vi "prova.vi"() -> ()   [LabVIEW 2021]
uses:
  <vilib>/MakerHub/LINX/Public/Peripherals/Analog/Analog Read 1 Chan.vi
  <vilib>/MakerHub/LINX/Public/Peripherals/Analog/Analog Read N Chans.vi
  <vilib>/MakerHub/LINX/Private/Local IO/LinxAnalogRead.vi
  <vilib>/MakerHub/LINX/Public/Utilities/Check Channel.vi
  <vilib>/Utility/file.llb/Write Delimited Spreadsheet (DBL).vi
  <vilib>/MakerHub/LINX/Public/Utilities/Open Serial.vi
  <vilib>/MakerHub/LINX/Public/Sensors/Motion/Servo/Servo Open One Channel.vi
  <vilib>/MakerHub/LINX/Public/Sensors/Motion/Servo/Servo Set Pulse Width One Channel.vi
  <vilib>/MakerHub/LINX/Private/Utilties/Generate Error.vi
  <vilib>/MakerHub/LINX/Public/Sensors/Motion/Servo/Servo Close One Channel.vi
  <vilib>/Utility/file.llb/Read Delimited Spreadsheet (DBL).vi
  <vilib>/MakerHub/LINX/LMH-LINX.lvlib
  <vilib>/MakerHub/LINX/Public/Sensors/Motion/Servo/Servo.lvlib
panel:
  out "Average":dbl[](array[numeric])
  out "Min. Wert":dbl
  out "Max. Wert":dbl
  out "all rows":dbl[][](array[numeric]) caption="Alle Zeilen"
  in  "Retrieve":bool
  in  "Dateipfad (Dialog verwenden)":path=path "C:/Users/Lucas Gomes/Documents/teste"
  in  "Button Channel":u8=2
  in  "Temp Channel":u8
  in  "Servo Channel":u8=3
  in  "VISA-Referenz (Eingang)":refnum<visa-resource-name>="COM3"
  in  "Stopp-Schaltfläche":bool
  out "Thermometer":dbl(slide) scale=0.0..100.0
  out "Signalverlaufsdiagramm 2":dbl(graph)
  # "5"
  # "Past data"
  # "Configurations"
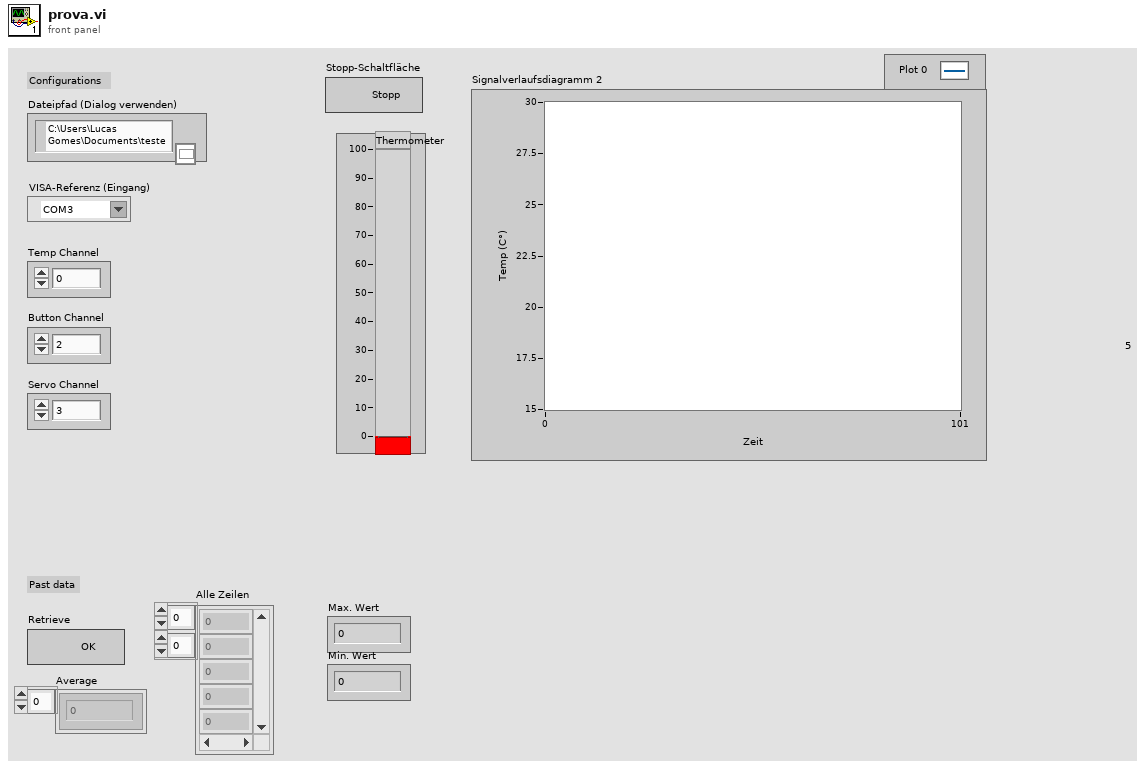
[diagram p1: front panel]
types:
  T1 = typedef "LMH-LINX.lvlib/LINX Ref.ctl" = cluster{"IO":T2, "Interface":T3, "LINX Device Config":T4}
  T2 = typedef "LMH-LINX.lvlib/Platform.ctl" = enum16{"Remote", "Local"}
  T3 = typedef "LMH-LINX.lvlib/Interface.ctl" = enum16{"Serial", "TCP"}
  T4 = typedef "LMH-LINX.lvlib/Device.lvlib/LINX Device Config.ctl" = cluster{"Interface":T3, "COM Port":refnum<visa-resource-name>, "TCP Configuration":T5, "Device Family":u8, "Device ID":u8, "Device Name":string, "TCP Ref":refnum<k5>, "Channels":T6}
  T5 = typedef "LMH-LINX.lvlib/Device.lvlib/TCP Config.ctl" = cluster{"IP Address":string, "Port":u16}
  T6 = typedef "LMH-LINX.lvlib/Channels.ctl" = cluster{"DI":u8[], "DO":u8[], "AI":u8[], "AO":u8[], "PWM":u8[], "QE":u8[], "UART":u8[], "I2C 2":u8[], "SPI":u8[], "CAN":u8[], "Servo":u8[], "AI Ref (V)":dbl, "AI Resolution (Bits)":u8, "AO Ref (V)":dbl, "AO Resolution (Bits)":u8}
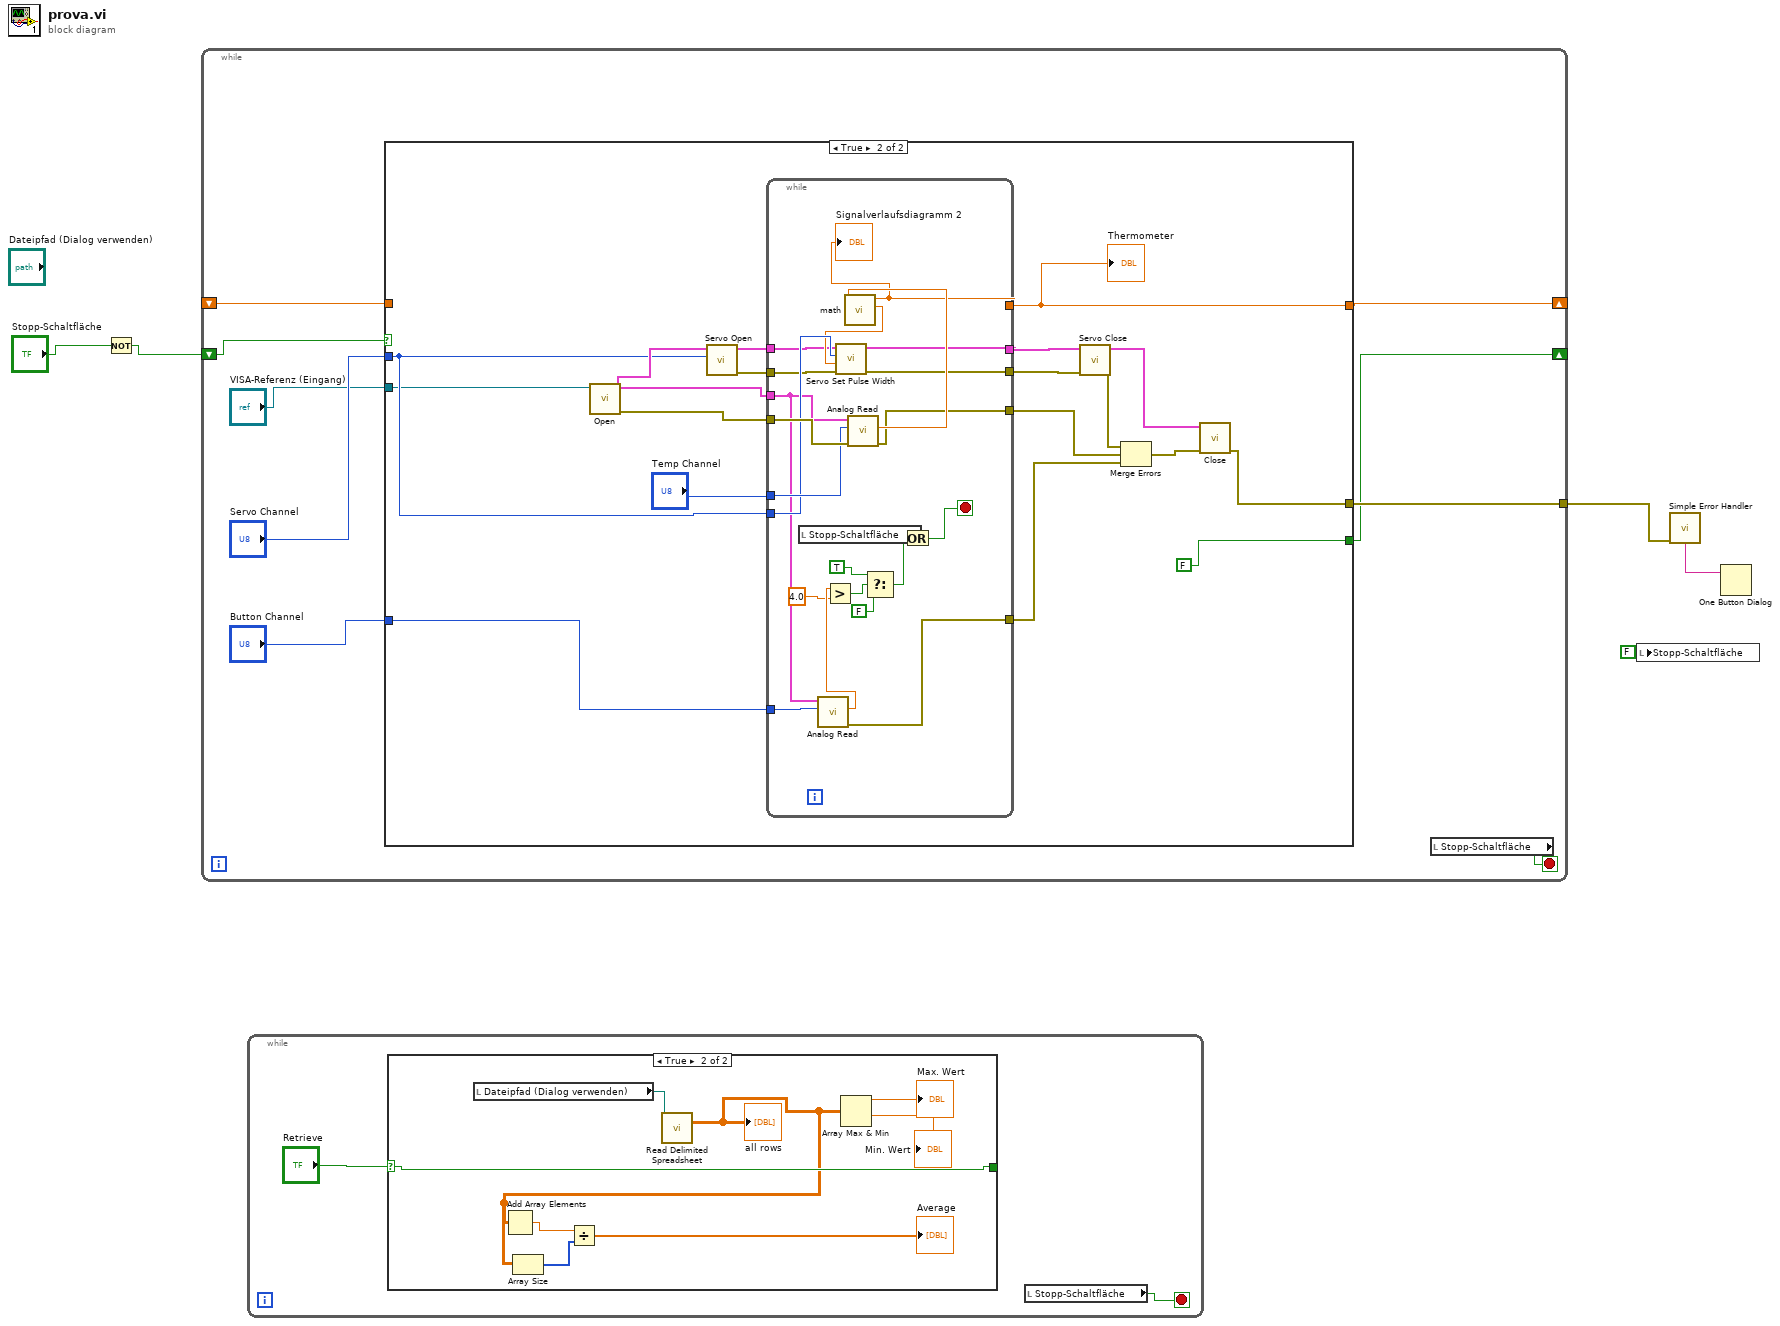
[diagram p0: block diagram]
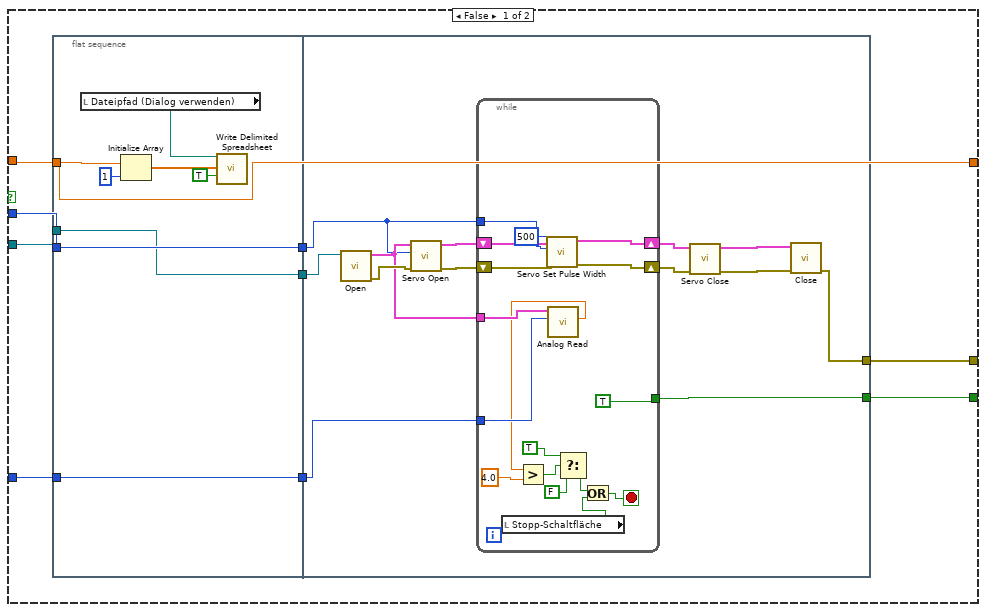
[diagram p3: hidden frame]
diagram:
  n1 = Not(x="Stopp-Schaltfläche") -> (.not. x?=w5:bool)
  n2 = while {
    shift-right: [w6] -> _
    shift-left: w5 -> [w13]
    shift-right: [w12] -> _
    shift-left: _ -> [w11]
    tunnel: [w7] -> w2
    stop <- w14 stop-if-true
    n3 = case shown="True" w13 {
      tunnel: [w22 FALSE] -> w6
      tunnel: [w23 w67] -> w12
      tunnel: w11 -> [w23 _]
      tunnel: "Button Channel" -> [w18 w66]
      tunnel: "Servo Channel" -> [w20 w65]
      tunnel: "VISA-Referenz (Eingang)" -> [w16 w64]
      tunnel: [w15 w63] -> w7
      frame False {
        n4 = flat-sequence {
          tunnel: w23 -> [w28]
          tunnel: [w27] -> w21
          tunnel: w20 -> [w27]
          tunnel: [w26] -> w19
          tunnel: w18 -> [w26]
          tunnel: [w25] -> w17
          tunnel: w16 -> [w25]
          tunnel: [w32] -> w22
          tunnel: w21 -> [w36]
          tunnel: w19 -> [w35]
          tunnel: w17 -> [w34]
          tunnel: [w33] -> w15
          frame #0 {
            n5 = local read "Dateipfad (Dialog verwenden)"() -> (w24:path)
            n6 = Initialize Array(w28, 1 ("Dimensionsgröße")) -> (w29:dbl[])
            n7 = call-poly <vilib>:"Write Delimited Spreadsheet.vi"("file path (dialog if empty)"=w24, "1D data"=w29, "append to file? (new file:F)"=TRUE) -> ()  [unwired: 11 in, 2 out]
          }
          frame #1 {
            n8 = call-poly <vilib>:"Open.vi"("Serial Port"=w34) -> ("Error Out"=w41:errorcluster, "LINX Resource"=w37:T1)  [unwired: 8 in, 1 out]
            n9 = call-poly <vilib>:"Servo Open.vi"("Error In"=w41, "Servo Channel"=w36, "LINX Resource"=w37) -> ("Error Out"=w40:errorcluster, "LINX Resource"=w44:T1)  [unwired: 7 in]
            n10 = while {
              tunnel: w37 -> [w57]
              tunnel: [TRUE] -> w32
              tunnel: w36 -> [w56]
              tunnel: w35 -> [w55]
              shift-right: [w60] -> w43
              shift-left: w44 -> [w61]
              shift-right: [w58] -> w39
              shift-left: w40 -> [w59]
              stop <- w48 stop-if-true
              n11 = local read "Stopp-Schaltfläche"() -> (w47:bool)
              n12 = call-poly <vilib>:"Servo Set Pulse Width.vi"("Error In"=w59, "Pulse Width (uS)"=u16 500, "Servo Channel"=w56, "LINX Resource"=w61) -> ("Error Out"=w58:errorcluster, "LINX Resource"=w60:T1)  [unwired: 6 in]
              n13 = call-poly <vilib>:"Analog Read.vi"("Analog Channel"=w55, "LINX Resource"=w57) -> ("Voltage"=w49:dbl)  [unwired: 6 in, 3 out]
              n14 = Greater?(x=w49, y=4.0) -> (0:w51:bool)
              n15 = Select(t=TRUE, s=w51, f=FALSE) -> (s? t:f=w46:bool)
              n16 = Or(x=w46, y=w47) -> (x .or. y?=w48:bool)
            }
            n17 = call-poly <vilib>:"Servo Close.vi"("Error In"=w39, "LINX Resource"=w43) -> ("Error Out"=w38:errorcluster, "LINX Resource"=w42:T1)  [unwired: 8 in]
            n18 = call <vilib>:"Close.vi"("Error In"=w38, "LINX Resource"=w42) -> ("Error Out"=w33:errorcluster)  [unwired: 9 in]
          }
        }
      }
      frame True {
        n19 = call-poly <vilib>:"Open.vi"("Serial Port"=w64) -> ("Error Out"=w78:errorcluster, "LINX Resource"=w79:T1)  [unwired: 8 in, 1 out]
        n20 = call-poly <vilib>:"Servo Open.vi"("Servo Channel"=w65, "LINX Resource"=w79) -> ("Error Out"=w76:errorcluster, "LINX Resource"=w75:T1)  [unwired: 8 in]
        n21 = while {
          tunnel: w79 -> [w89]
          tunnel: w78 -> [w101]
          tunnel: "Temp Channel" -> [w100]
          tunnel: w65 -> [w98]
          tunnel: [w91] -> w67
          tunnel: w76 -> [w96]
          tunnel: w75 -> [w95]
          tunnel: [w94] -> w73
          tunnel: [w93] -> w74
          tunnel: [w92] -> w72
          tunnel: w66 -> [w88]
          tunnel: [w87] -> w68
          stop <- w86 stop-if-true
          n22 = local read "Stopp-Schaltfläche"() -> (w90:bool)
          n23 = call-poly <vilib>:"Analog Read.vi"("Analog Channel"=w88, "LINX Resource"=w89) -> ("Error Out"=w87:errorcluster, "Voltage"=w81:dbl)  [unwired: 6 in, 2 out]
          n24 = Greater?(x=w81, y=4.0) -> (0:w82:bool)
          n25 = call-poly <vilib>:"Analog Read.vi"("Error In"=w101, "Analog Channel"=w100, "LINX Resource"=w89) -> ("Error Out"=w92:errorcluster, "Voltage"=w99:dbl)  [unwired: 5 in, 2 out]
          n26 = call "math.vi"("Voltage"=w99) -> ("Numerisch 2"=w97:dbl, "Numerisch"=w91:dbl)  [unwired: 9 in]
          "Signalverlaufsdiagramm 2" <- w91
          n27 = call-poly <vilib>:"Servo Set Pulse Width.vi"("Error In"=w96, "Pulse Width (uS)"=w97, "Servo Channel"=w98, "LINX Resource"=w95) -> ("Error Out"=w94:errorcluster, "LINX Resource"=w93:T1)  [unwired: 6 in]
          n28 = Select(t=TRUE, s=w82, f=FALSE) -> (s? t:f=w85:bool)
          n29 = Or(x=w90, y=w85) -> (x .or. y?=w86:bool)
        }
        "Thermometer" <- w67
        n30 = call-poly <vilib>:"Servo Close.vi"("Error In"=w73, "LINX Resource"=w74) -> ("Error Out"=w70:errorcluster, "LINX Resource"=w69:T1)  [unwired: 8 in]
        n31 = Merge Errors(w70, w72, w68) -> (w71:errorcluster)
        n32 = call <vilib>:"Close.vi"("Error In"=w71, "LINX Resource"=w69) -> ("Error Out"=w63:errorcluster)  [unwired: 9 in]
      }
    }
    n33 = local read "Stopp-Schaltfläche"() -> (w14:bool)
  }
  n34 = while {
    stop <- w103 stop-if-true
    n35 = case shown="True" "Retrieve" {
      selector: "Retrieve" -> [w104 w111]
      tunnel: [w104 w111] -> _
      frame False {
      }
      frame True {
        n36 = local read "Dateipfad (Dialog verwenden)"() -> (w112:path)
        n37 = call-poly <vilib>:"Read Delimited Spreadsheet.vi"("file path (dialog if empty)"=w112) -> ("all rows"=w108:dbl[][])  [unwired: 9 in, 5 out]
        "all rows" <- w108
        n38 = Add Array Elements(numeric array=w108) -> (sum=w107:dbl)
        n39 = Array Size(array=w108) -> (size(s)=w106:i32[])
        n40 = Divide(x=w107, y=w106) -> (x/y=→"Average":dbl[])
        n41 = Array Max & Min(array=w108) -> (max value=→"Max. Wert":dbl, min value=→"Min. Wert":dbl)  [unwired: 2 out]
      }
    }
    n42 = local read "Stopp-Schaltfläche"() -> (w103:bool)
  }
  n43 = local write "Stopp-Schaltfläche"(FALSE ("OK-Schaltfläche")) -> ()
  n44 = call <vilib>:"Simple Error Handler.vi"("error in (no error)"=w2) -> ("message"=w3:string)  [unwired: 4 in, 4 out]
  n45 = One Button Dialog(message=w3) -> ()  [unwired: 1 in, 1 out]
